vi "initialize_queue.vi"(8 "error in (no error)":errorcluster, 11 "state":T1=enum."(qsm) initialize") -> (0 "error out":errorcluster, 3 "queue out":refnum<queue>)   [LabVIEW 2025]
uses:
  type defs/state.ctl
  type defs/task.ctl
panel:
  # "initialize_queue"
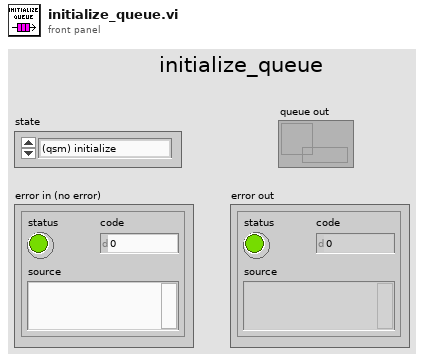
[diagram p1: front panel]
types:
  T1 = typedef "state.ctl" = enum16{"(qsm) schedule", "(qsm) initialize", "(qsm) release", "(qsm) clean up", "(qsm) shutdown", "(HW) initialize", "((HW)) clean up", "((HW)) update ports", "(image) get", "(image) analyze", "(image) overlay", "(image) show", "save image", "state A", "state B", "state C", "state D", "state E", "state F", "state G", "state H"}
  T2 = typedef "task.ctl" = T1[]
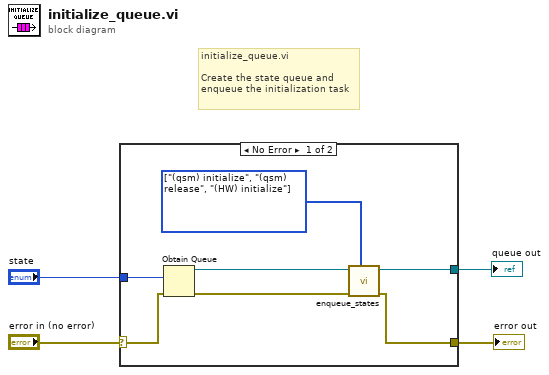
[diagram p0: block diagram]
diagram:
  # "initialize_queue.vi\n\nCreate the state queue and\nenqueue the initialization task"
  n1 = case shown="No Error" "error in (no error)" {
    selector: "error in (no error)" -> [w8 w12]
    tunnel: [w7 w12] -> w3
    tunnel: [w9 _] -> w2
    tunnel: "state" -> [w5 _]
    frame No Error {
      w6 = T2 [enum."(qsm) initialize", enum."(qsm) release", enum."(HW) initialize"] items=["(qsm) schedule", "(qsm) initialize", "(qsm) release", "(qsm) clean up", "(qsm) shutdown", "(HW) initialize", "((HW)) clean up", "((HW)) update ports", "(image) get", "(image) analyze", "(image) overlay", "(image) show", "save image", "state A", "state B", "state C", "state D", "state E", "state F", "state G", "state H"] ("task")
      n2 = Obtain Queue(element data type=w5, error in (no error)=w8) -> (queue out=w11:refnum<queue>, error out=w10:errorcluster)  [unwired: 3 in, 1 out]
      n3 = call "enqueue_states.vi"("task"=w6, "error in"=w10, "queue in"=w11) -> ("error out"=w7:errorcluster, "queue out"=w9:refnum<queue>)  [unwired: 7 in]
    }
    frame Error {
    }
  }
  "error out" <- w3
  "queue out" <- w2
